vi "Arcade Drive.vi"() -> ()   [LabVIEW 2025]
doc: "Arcade Drive Example\n\nThis example shows arcade drive using the joystick to update motor speeds.\n\nThis example expects a USB cable connected from your development PC to the Type B USB Jack (next to the power input) on the roboRIO.\n\nThis example requires the Driver Station to be running with Teleoperated Enabled."
uses:
  <vilib>/Rock Robotics/SystemInterfaces/DIO/FPGA_DIOPWMChannel.ctl
  <vilib>/Rock Robotics/WPI/Joystick/WPI_JoystickDeviceEnum.ctl
  <vilib>/Rock Robotics/WPI/RobotDrive/WPI_RobotDriveOpen2MotorWithTalon.vi
  <vilib>/Rock Robotics/WPI/RobotDrive/WPI_RobotDriveArcadeDrive_Standard(NoSaturation).vi
panel:
  in  "Joystick":T1
  in  "Left Motor (PWM channel)":T2
  in  "Right Motor (PWM channel)":T2=enum."PWM 1"
  in  "stop":bool
  # "Set these inputs before running."
  # "This example requires the Driver Station to be running with Teleoperated Enabled."
  # "PWM cables"
  # "This shows wiring for Talon speed controllers.  The wiring is similar for other motor controllers.  If you change the controller type, you must also select the appropriate instance of the Motor Open VI on the diagram."
  # "Power\nTerminals"
  # "Motor\nTerminals"
  # "+"
  # "+"
  # "M"
  # "B"
  # "Power\nTerminals"
  # "Motor\nTerminals"
  # "+"
  # "+"
  # "M"
  # "B"
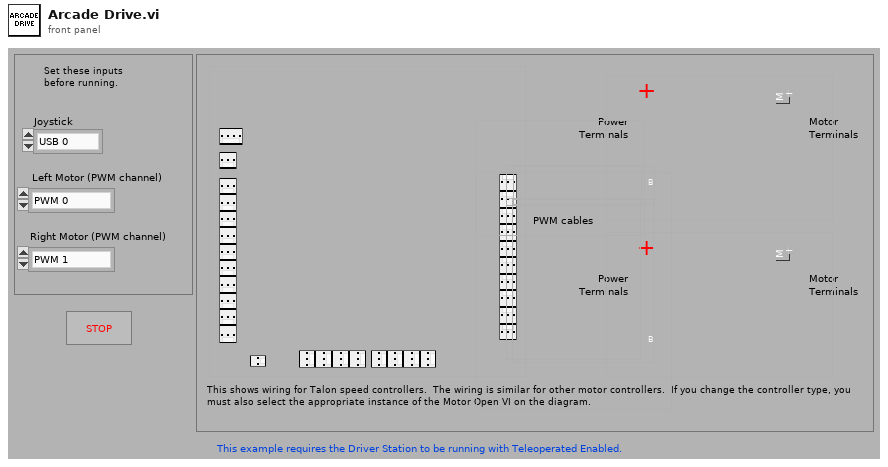
[diagram p1: front panel]
types:
  T1 = typedef "WPI_JoystickDeviceEnum.ctl" = enum16{"USB 0", "USB 1", "USB 2", "USB 3", "USB 4", "USB 5"}
  T2 = typedef "FPGA_DIOPWMChannel.ctl" = enum8{"PWM 0", "PWM 1", "PWM 2", "PWM 3", "PWM 4", "PWM 5", "PWM 6", "PWM 7", "PWM 8", "PWM 9", "PWM MXP 0", "PWM MXP 1", "PWM MXP 2", "PWM MXP 3", "PWM MXP 4", "PWM MXP 5", "PWM MXP 6", "PWM MXP 7", "PWM MXP 8", "PWM MXP 9", "Invalid"}
  T3 = typedef "WPI_JoystickDevRef.ctl" = cluster{"Device":T1}
  T4 = typedef "WPI_RobotDriveDevRef.ctl" = cluster{"DevStatus":errorcluster, "Motors[]":T5[], "Square Inputs":bool, "Max Output":dbl}
  T5 = typedef "WPI_MotorControlDeviceRef.ctl" = cluster{"DeviceStatus":errorcluster, "Type":T6, "PWM":cluster{"PWM Channel":T2, "DeadBand":T7}, "CAN":cluster{"Device Number":u8, "SetOutput VI Ref":variant, "GetOutput VI Ref":variant, "Enable VI Ref":variant, "Disable VI Ref":variant, "Data":variant}, "Invert":bool, "DIO PWM":cluster{"PWM \"Enable\" Channel":T2, "DIOChannel":T8, "PWM Rate":dbl}}
  T6 = typedef "WPI_MotorControlType.ctl" = enum16{"PWM", "CAN", "DIO PWM"}
  T7 = typedef "WPI_PWMDeadband.ctl" = cluster{"Name":string, "maxPositivePwm":i32, "minPositivePwm":i32, "centerPwm":i32, "maxNegativePwm":i32, "minNegativePwm":i32, "angularRange":u16}
  T8 = typedef "FPGA_DIOChannel.ctl" = enum8{"DIO 0", "DIO 1", "DIO 2", "DIO 3", "DIO 4", "DIO 5", "DIO 6", "DIO 7", "DIO 8", "DIO 9", "DIO MXP 0", "DIO MXP 1", "DIO MXP 2", "DIO MXP 3", "DIO MXP 4", "DIO MXP 5", "DIO MXP 6", "DIO MXP 7", "DIO MXP 8", "DIO MXP 9", "DIO MXP 10", "DIO MXP 11", "DIO MXP 12", "DIO MXP 13", "DIO MXP 14", "DIO MXP 15", "SPI Port CS1", "SPI Port CS2", "SPI Port CS3", "SPI Port MISO", "SPI Port MOSI", "Invalid"}
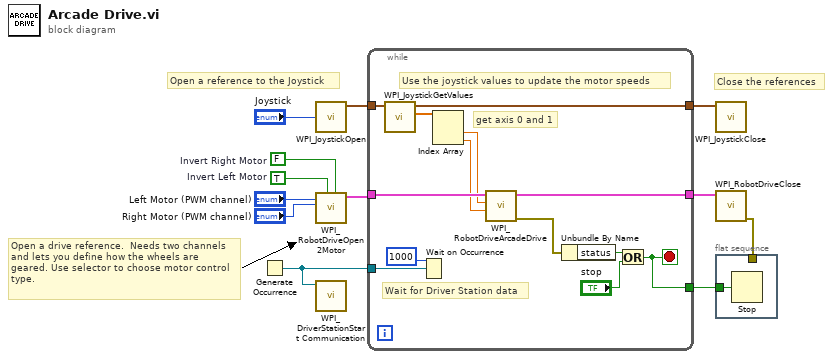
[diagram p0: block diagram]
diagram:
  w6 = FALSE  # Invert Right Motor
  w7 = TRUE  # Invert Left Motor
  # "Open a reference to the Joystick"
  # "Close the references"
  # "Open a drive reference.  Needs two channels and lets you define how the wheels are geared. Use selector to choose motor control type."
  n1 = Generate Occurrence() -> (w8:refnum<k4>)
  n2 = call <vilib>:"WPI_JoystickOpen.vi"("JoystickDevice"="Joystick") -> ("JoystickDevRef"=w4:T3)  [unwired: 10 out]
  n3 = call-poly <vilib>:"WPI_RobotDriveOpen2Motor.vi"("Right Motor Inverted"=w6, "Left Motor Inverted"=w7, "Right Motor"="Right Motor (PWM channel)", "Left Motor"="Left Motor (PWM channel)") -> ("RobotDriveDevRef"=w10:T4)  [unwired: 1 in, 6 out]
  n4 = call <vilib>:"WPI_DriverStationStart Communication.vi"("occurrence"=w8) -> ()  [unwired: 2 in, 9 out]
  n5 = while {
    tunnel: w10 -> [w22]
    tunnel: [w21] -> w9
    tunnel: [w17] -> w2
    tunnel: w8 -> [w25]
    tunnel: w4 -> [w23]
    tunnel: [w16] -> w3
    stop <- w17 stop-if-true
    # "get axis 0 and 1"
    # "Wait for Driver Station data"
    # "Use the joystick values to update the motor speeds"
    n6 = call <vilib>:"WPI_JoystickGetValues.vi"("JoystickDevRef"=w23) -> ("Axes"=w15:dbl[], "JoystickDevRef"=w16:T3)  [unwired: 6 in, 3 out]
    n7 = Wait on Occurrence(2:w25, 3:1000 ("ms timeout (-1)")) -> ()  [unwired: 2 out]
    n8 = Index Array(array=w15) -> (element #1=w14:dbl, element #2=w13:dbl)  [unwired: 2 in]
    n9 = call-poly <vilib>:"WPI_RobotDriveArcadeDrive.vi"("Y axis value"=w13, "X axis value"=w14, "RobotDriveDevRef"=w22) -> ("error out"=w20:errorcluster, "RobotDriveDevRef"=w21:T4)  [unwired: 1 in, 6 out]
    n10 = Unbundle By Name(w20) -> ("status"=w19:bool)
    n11 = Or(x=w19, y="stop") -> (x .or. y?=w17:bool)
  }
  n12 = call <vilib>:"WPI_JoystickClose.vi"("JoystickDevRef"=w3) -> ()  [unwired: 11 out]
  n13 = call <vilib>:"WPI_RobotDriveClose.vi"("RobotDriveDevRef"=w9) -> ("error out"=w1:errorcluster)  [unwired: 1 in, 9 out]
  n14 = flat-sequence {
    tunnel: w2 -> [w26]
    tunnel: w1 -> [_]
    frame #0 {
      n15 = Stop(stop? (T)=w26) -> ()
    }
  }
